vi "MTM2_monitorCommand_applyBendingMode.vi"(8 "error in (no error)":errorcluster, 11 "command_applyBendingMode_Ctl":T1={"bendingModeNbr[32]"=[0, 0, 0, 0, 0, 0, 0, 0, 0, 0, 0, 0, 0, 0, 0, 0, 0, 0, 0, 0, 0, 0, 0, 0, 0, 0, 0, 0, 0, 0, 0, 0], "bendingModeValue[32]"=[0.0, 0.0, 0.0, 0.0, 0.0, 0.0, 0.0, 0.0, 0.0, 0.0, 0.0, 0.0, 0.0, 0.0, 0.0, 0.0, 0.0, 0.0, 0.0, 0.0, 0.0, 0.0, 0.0, 0.0, 0.0, 0.0, 0.0, 0.0, 0.0, 0.0, 0.0, 0.0]}) -> (0 "error out":errorcluster, 2 "function return":i32, 3 "command_applyBendingMode_Ctl out":T1)   [LabVIEW 2018, in "SALLV_MTM2.lvlib"]
doc: "int MTM2_shm_monitorCommand_applyBendingModeLV(MTM2_command_applyBendingModeLV *command_applyBendingMode_Ctl );"
uses:
  SALLV_MTM2.lvlib
  DataTypes/command_applyBendingMode.ctl
  SALLV_MTM2.so
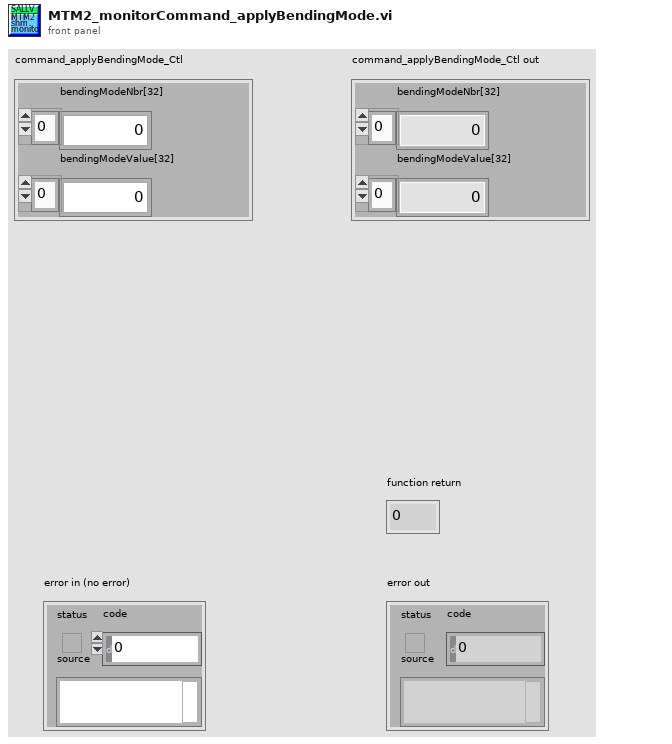
[diagram p1: front panel]
types:
  T1 = typedef "SALLV_MTM2.lvlib/command_applyBendingMode.ctl" = cluster{"bendingModeNbr[32]":i16[], "bendingModeValue[32]":dbl[]}
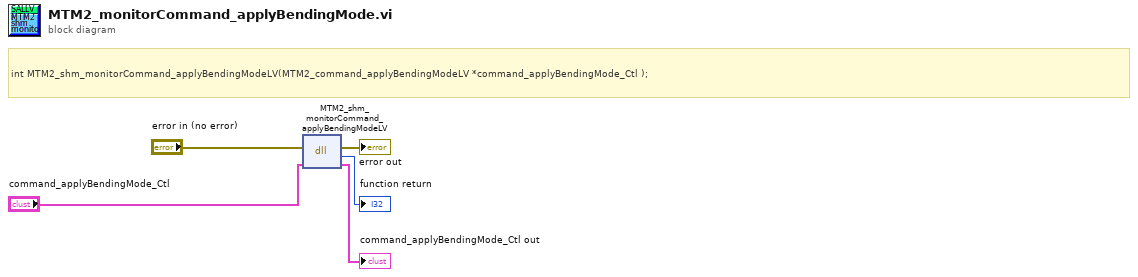
[diagram p0: block diagram]
diagram:
  # "int MTM2_shm_monitorCommand_applyBendingModeLV(MTM2_command_applyBendingModeLV *command_applyBendingMode_Ctl );"
  n1 = dll-call lib="home/ttsai/Document/salApiMTM2/SALLV_MTM2/SALLV_MTM2.*" fn="MTM2_shm_monitorCommand_applyBendingModeLV"(error in="error in (no error)", "command_applyBendingMode_Ctl"="command_applyBendingMode_Ctl") -> (error out=→"error out":errorcluster, →"function return":i32, "command_applyBendingMode_Ctl"=→"command_applyBendingMode_Ctl out":T1)  [unwired: 2 in, 1 out]
